vi "Read Temperature Log.vi"(0 "file path":path) -> (1 "Temperature Log":dbl[](array[numeric]), 2 "error out":errorcluster)   [LabVIEW 2010]
uses:
  SupportVIs.llb/TS_RT-Open/Create/Replace File.vi
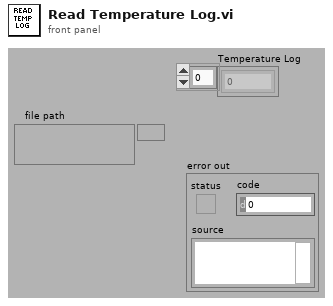
[diagram p1: front panel]
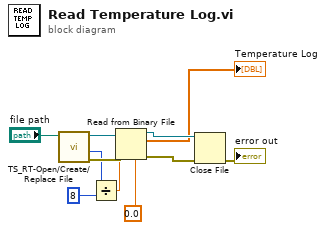
[diagram p0: block diagram]
diagram:
  n1 = call "TS_RT-Open/Create/Replace File.vi"("file path"="file path") -> ("error out"=w11:errorcluster, "file size (bytes)"=w7:i32, "refnum"=w9:refnum<file>)  [unwired: 5 in, 3 out]
  n2 = Divide(x=w7, y=8) -> (x/y=w5:dbl)
  n3 = Read from Binary File(5:0.0, 8:w11, 10:w5, 11:w9) -> (0:w10:errorcluster, 2:→"Temperature Log":dbl[], 3:w8:refnum<file>)  [unwired: 3 out]
  n4 = Close File(refnum=w8, error in=w10) -> (error out=→"error out":errorcluster)  [unwired: 1 out]
